vi "Configure Acquisition Record.vi"(0 "CS++Scope":refnum<class "CS++Scope.lvclass">, 5 "time per record (1.0E-3 s)":dbl[unit]=0.001 format="%^.2e", 7 "min record length (100 samples)":i32=100, 9 "acquisition start time (0.0 s)":dbl[unit] format="%.3f", 11 "error in (no error)":errorcluster) -> (4 "CS++Scope out":refnum<class "CS++Scope.lvclass">, 15 "error out":errorcluster)   [LabVIEW 2013, in "CS++Scope.lvlib" / "CS++Scope.lvclass"]
doc: "This VI configures the most commonly configured properties of the oscilloscope acquisition subsystem. These properties are the time per record, minimum record length, and the acquisition start time."
uses:
  CS++Scope.lvclass
  CSPP_Core/Classes/CS++ProcessVariables/ProcessVariable/PV.lvclass
  PV-Enum.ctl
  CS++Scope.lvclass/CS++Scope.ctl
  CSPP_Core/Classes/CS++ProcessVariables/PVConnection/PVConnection.lvclass
  CSPP_Core/Classes/CS++ProcessVariables/ProcessVariable/PV.lvclass/PV.ctl
  CSPP_Core/Classes/CS++ProcessVariables/ProcessVariable/Write Data.vi
  CSPP_Core/Classes/CS++ProcessVariables/ProcessVariable/Write Timestamp.vi
  CSPP_Core/Classes/CS++ProcessVariables/ProcessVariable/Write Quality.vi
  CSPP_Core/Classes/CS++ProcessVariables/ProcessVariable/Write status.vi
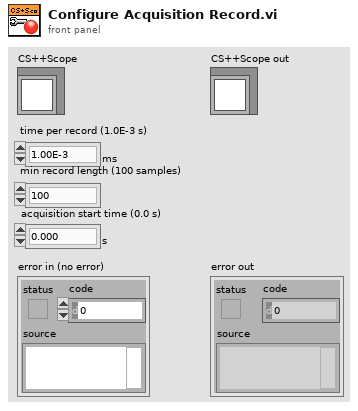
[diagram p1: front panel]
types:
  T1 = typedef "CS++Scope.lvlib/CS++Scope.lvclass/PV-Enum.ctl" = enum16{"ActualSampleRate", "TimePerRecord", "AcquisitionStartTime", "TriggerLevel", "GlitchWidth", "LowReference", "MidReference", "HighReference", "RuntLowThreshold", "RuntHighThreshold", "TriggerHoldoff", "WidthLowThreshold", "WidthHighThreshold", "AcquisitionStatus", "ActualRecordLength", "ActualSampleMode", "ACLineTriggerSlope", "MinRecordLength", "AcquisitionType", "TriggerSlope", "GlitchCondition", "GlitchPolarity", "InterpolationMethod", "NumberOfAverages", "NumberOfEnvelopes", "TriggerType", "TriggerCoupling", "TriggerModifier", "TVLineNumber", "TVEvent", "TVTriggerPolarity", "TVSignalFormat", "WidthCondition", "WidthPolarity", "MeasurementDone", "ContinousAcquisition", "TriggerSource", "Waveform"}
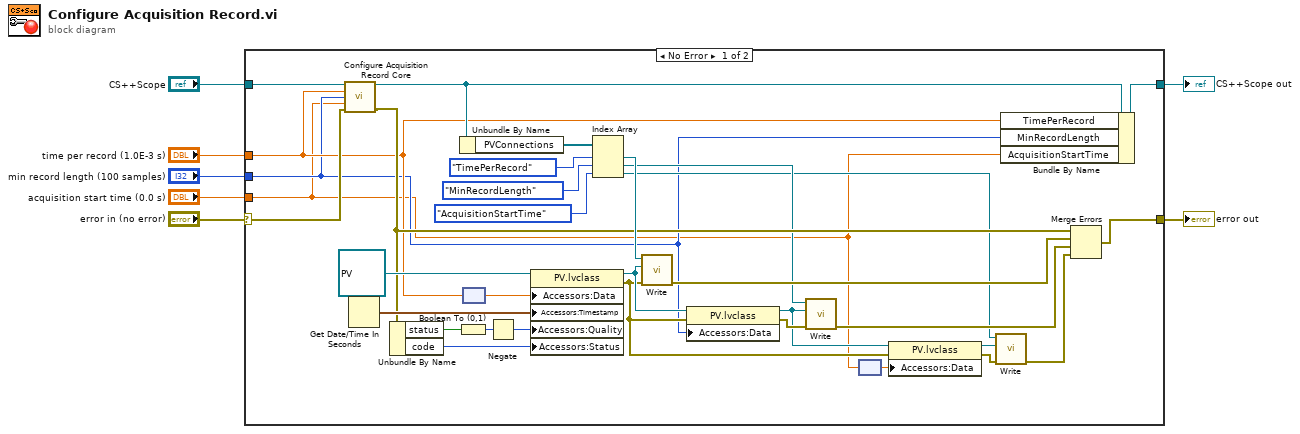
[diagram p0: block diagram]
diagram:
  n1 = case shown="No Error" "error in (no error)" {
    selector: "error in (no error)" -> [w26 w42]
    tunnel: [w29 w42] -> w6
    tunnel: [w30 w41] -> w2
    tunnel: "CS++Scope" -> [w28 w41]
    tunnel: "time per record (1.0E-3 s)" -> [w12 _]
    tunnel: "min record length (100 samples)" -> [w11 _]
    tunnel: "acquisition start time (0.0 s)" -> [w9 _]
    frame No Error {
      n2 = call-dynamic "Configure Acquisition Record Core.vi"("CS++Scope"=w28, "time per record (1.0E-3 s)"=w12, "min record length (100 samples)"=w11, "acquisition start time (0.0 s)"=w9, "error in (no error)"=w26) -> ("CS++Scope out"=w27:refnum<class "CS++Scope.lvclass">, "error out"=w25:errorcluster)  [unwired: 9 in]
      n3 = Get Date/Time In Seconds() -> (seconds since 1Jan1904=w35:timestamp)
      n4 = Unbundle By Name(w25) -> ("status"=w38:bool, "code"=w39:i32)
      n5 = Boolean To (0,1)(Boolean=w38) -> (0, 1=w37:i16)
      n6 = Unbundle By Name(w27) -> ("PVConnections"=w34:refnum<class "PVConnection.lvclass">[])
      n7 = node(w12) -> (w10:dbl)
      n8 = Negate(x=w37) -> (-x=w36:i16)
      n9 = property class="PV.lvclass"(reference=refnum<class "PV.lvclass"> refnum ("CS++ProcessVariables.lvlib:PV.lvclass"), "Accessors:Data"=w10, "Accessors:Timestamp"=w35, "Accessors:Quality"=w36, "Accessors:Status"=w39) -> (reference out=w20:refnum<class "PV.lvclass">, error out=w16:errorcluster)  [unwired: 1 in]
      n10 = Index Array(array=w34, index #1=PV-Enum."TimePerRecord" ("PV-Enum"), index #2=PV-Enum."MinRecordLength" ("PV-Enum"), index #3=PV-Enum."AcquisitionStartTime" ("PV-Enum")) -> (element #1=w32:refnum<class "PVConnection.lvclass">, element #2=w18:refnum<class "PVConnection.lvclass">, element #3=w14:refnum<class "PVConnection.lvclass">)
      n11 = call-dynamic "Write.vi"("error in (no error)"=w16, "PV"=w20, "PVConnection in"=w32) -> ("error out"=w31:errorcluster)  [unwired: 7 in, 1 out]
      n12 = property class="PV.lvclass"(reference=w20, error in=w16, "Accessors:Data"=w11) -> (reference out=w17:refnum<class "PV.lvclass">, error out=w19:errorcluster)
      n13 = call-dynamic "Write.vi"("error in (no error)"=w19, "PV"=w17, "PVConnection in"=w18) -> ("error out"=w22:errorcluster)  [unwired: 7 in, 1 out]
      n14 = node(w9) -> (w8:dbl)
      n15 = property class="PV.lvclass"(reference=w17, error in=w16, "Accessors:Data"=w8) -> (reference out=w15:refnum<class "PV.lvclass">, error out=w13:errorcluster)
      n16 = call-dynamic "Write.vi"("error in (no error)"=w13, "PV"=w15, "PVConnection in"=w14) -> ("error out"=w21:errorcluster)  [unwired: 7 in, 1 out]
      n17 = Bundle By Name(cluster=w27, "TimePerRecord"=w12, "MinRecordLength"=w11, "AcquisitionStartTime"=w9) -> (w30:refnum<class "CS++Scope.lvclass">)
      n18 = Merge Errors(w25, w31, w22, w21) -> (w29:errorcluster)
    }
    frame Error {
    }
  }
  "error out" <- w6
  "CS++Scope out" <- w2
